vi "Day04-05_지진 계측기 프로젝트_생산자,소비자.vi"() -> ()   [LabVIEW 2021]
uses:
  <vilib>/numeric/Random Number (Range) DBL.vi
panel:
  out "웨이브폼 차트":dbl(graph)
  in  "알람 리셋":bool
  out "LED":bool
  in  "정지":bool
  in  "감지 시작":bool
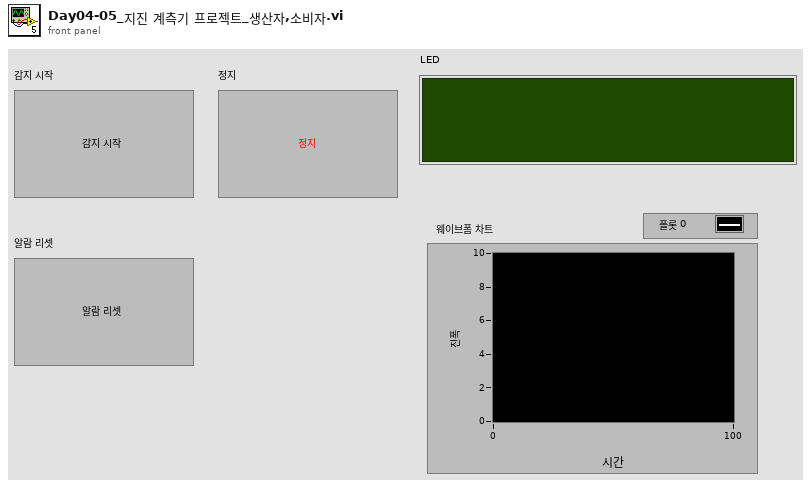
[diagram p1: front panel]
types:
  T1 = typedef "지진 계측기 상태 열거형 상수.ctl" = enum16{"초기화", "대기", "감지 시작", "알림 리셋", "정지"}
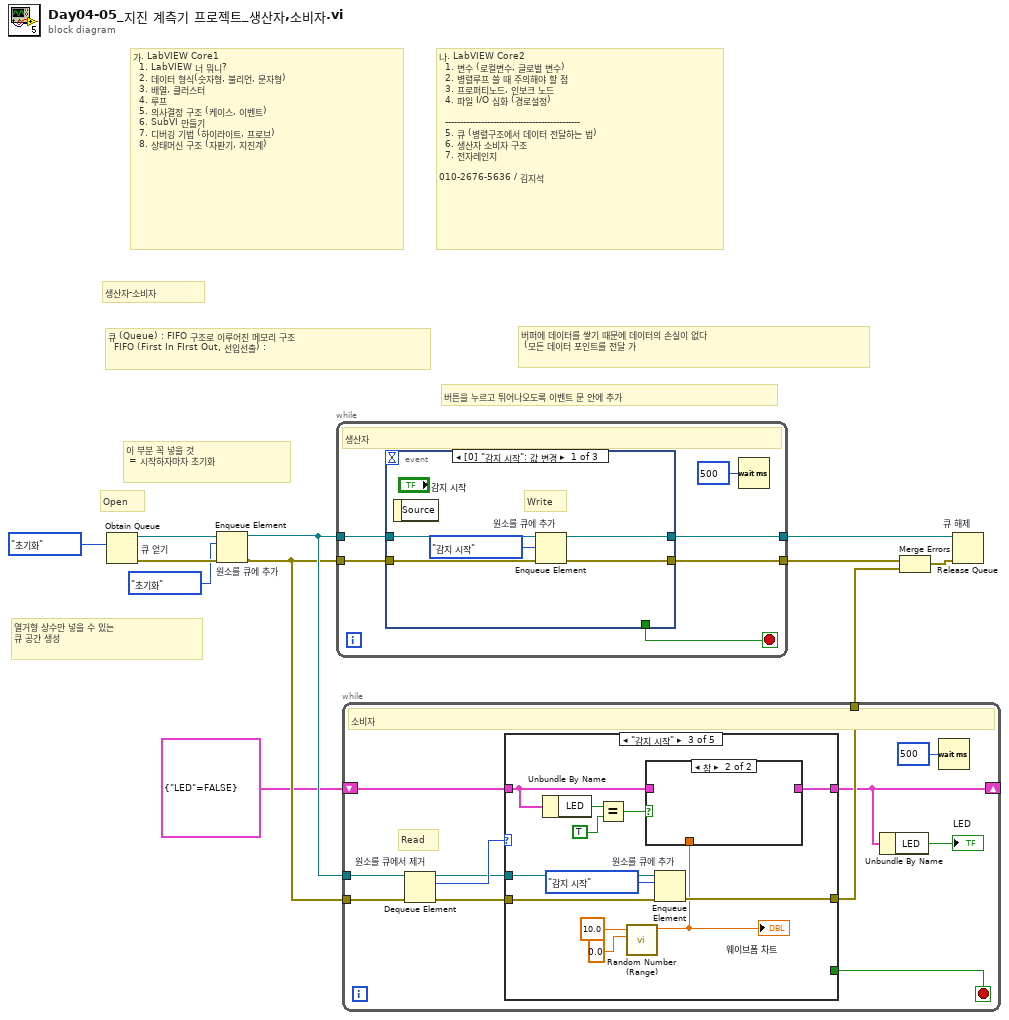
[diagram p0: block diagram]
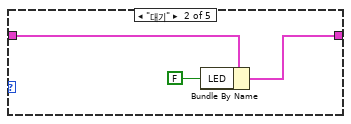
[diagram p3: hidden frame]
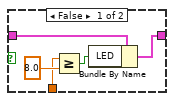
[diagram p4: hidden frame]
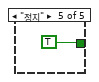
[diagram p6: hidden frame]
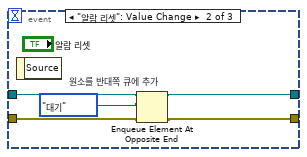
[diagram p7: hidden frame]
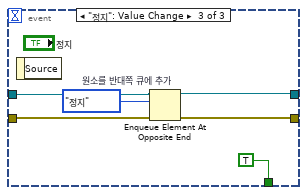
[diagram p8: hidden frame]
diagram:
  # "생산자-소비자"
  # "열거형 상수만 넣을 수 있는\n큐 공간 생성"
  # "이 부분 꼭 넣을 것\n = 시작하자마자 초기화"
  # "버튼을 누르고 튀어나오도록 이벤트 문 안에 추가"
  # "버퍼에 데이터를 쌓기 때문에 데이터의 손실이 없다\n (모든 데이터 포인트를 전달 가"
  # "Open"
  # "큐 (Queue) : FIFO 구조로 이루어진 메모리 구조\n  FIFO (First In FIrst Out, 선입선출) :"
  # "나. LabVIEW Core2\n  1. 변수 (로컬변수, 글로벌 변수)\n  2. 병렬루프 쓸 때 주의해야 할 점\n  3. 프로퍼티노드, 인보크 노드\n  4. 파일 I/O 심화 (경로설정)\n\n  ---------------------------------------------\n  5. 큐 (병렬구조에서 데이터 전달하는 법)\n  6. 생산자 소비자 구조\n  7. 전자레인지\n\n010-2676-5636 / 김지석"
  # "가. LabVIEW Core1\n  1. LabVIEW 너 뭐니?\n  2. 데이터 형식(숫자형, 불리언, 문자형)\n  3. 배열, 클러스터\n  4. 루프\n  5. 의사결정 구조 (케이스, 이벤트)\n  6. SubVI 만들기\n  7. 디버깅 기법 (하이라이트, 프로브)\n  8. 상태머신 구조 (자판기, 지진계)"
  n1 = Obtain Queue "큐 얻기"(element data type=지진_계측기_상태_열거형_상수."초기화") -> (queue out=w6:refnum<queue>, error out=w4:errorcluster)  [unwired: 4 in, 1 out]
  n2 = Enqueue Element "원소를 큐에 추가"(queue=w6, element=지진_계측기_상태_열거형_상수."초기화" ("원소"), error in (no error)=w4) -> (queue out=w5:refnum<queue>, error out=w3:errorcluster)  [unwired: 1 in, 1 out]
  n3 = while {
    tunnel: w5 -> [w17]
    tunnel: w3 -> [w16]
    tunnel: [w14] -> w8
    tunnel: [w13] -> w9
    stop <- w12 stop-if-true
    # "생산자"
    n4 = event shown="[0] \"감지 시작\": 값 변경" {
      selector: _ -> [_ _ _]
      dyn-events: _ -> [_ _ _]
      timeout: _ -> [_ _ _]
      tunnel: w17 -> [w22 w26 w30]
      tunnel: w16 -> [w19 w25 w31]
      tunnel: [w21 w27 w28] -> w14
      tunnel: [w20 w24 w32] -> w13
      tunnel: [_ _ TRUE] -> w12
      event "감지 시작": Value Change {
        # "Write"
        n5 = event-data() -> ()  [unwired: 1 in, 1 out]
        n6 = Enqueue Element "원소를 큐에 추가"(queue=w22, element=지진_계측기_상태_열거형_상수."감지 시작", error in (no error)=w19) -> (queue out=w21:refnum<queue>, error out=w20:errorcluster)  [unwired: 1 in, 1 out]
      }
      event "알람 리셋": Value Change {
        n7 = event-data() -> ()  [unwired: 1 in, 1 out]
        n8 = Enqueue Element At Opposite End "원소를 반대쪽 큐에 추가"(queue=w26, element=지진_계측기_상태_열거형_상수."대기", error in (no error)=w25) -> (queue out=w27:refnum<queue>, error out=w24:errorcluster)  [unwired: 1 in, 1 out]
      }
      event "정지": Value Change {
        n9 = event-data() -> ()  [unwired: 1 in, 1 out]
        n10 = Enqueue Element At Opposite End "원소를 반대쪽 큐에 추가"(queue=w30, element=지진_계측기_상태_열거형_상수."정지", error in (no error)=w31) -> (queue out=w28:refnum<queue>, error out=w32:errorcluster)  [unwired: 1 in, 1 out]
      }
    }
    n11 = Wait (ms)(milliseconds to wait=u32 500 ("대기 시간 (ms)")) -> ()  [unwired: 1 out]
  }
  n12 = while {
    tunnel: w3 -> [w44]
    tunnel: w5 -> [w43]
    tunnel: [w37] -> w10
    shift-right: [w34] -> _
    shift-left: cluster{"LED":bool} {"LED"=FALSE} -> [w35]
    stop <- w40 stop-if-true
    # "Read"
    # "소비자"
    n13 = Dequeue Element "원소를 큐에서 제거"(queue=w43, error in (no error)=w44) -> (queue out=w39:refnum<queue>, element=w41:T1, error out=w38:errorcluster)  [unwired: 1 in, 1 out]
    n14 = case shown="\"감지 시작\"" w41 {
      tunnel: [_ _ _ _ TRUE] -> w40
      tunnel: w39 -> [_ _ w59 _ _]
      tunnel: w38 -> [_ _ w58 _ _]
      tunnel: [_ _ w57 _ _] -> w37
      tunnel: w35 -> [_ w46 w49 _ _]
      tunnel: [_ w45 w53 _ _] -> w34
      frame "초기화", Default {
      }
      frame "대기" {
        n15 = Bundle By Name(cluster=w46, "LED"=FALSE) -> (w45:cluster{"LED":bool})
      }
      frame "감지 시작" {
        n16 = Unbundle By Name(w49) -> ("LED"=w54:bool)
        n17 = Equal?(x=w54, y=TRUE) -> (x = y?=w55:bool)
        n18 = call-poly <vilib>:"Random Number (Range).vi"("lower bound (0)"=0.0, "upper bound (100)"=10.0) -> ("number"=w48:dbl)  [unwired: 9 in]
        "웨이브폼 차트" <- w48
        n19 = case shown="참" w55 {
          tunnel: [w63 _] -> w53
          tunnel: w49 -> [w64 _]
          tunnel: w48 -> [w61 _]
          frame False {
            n20 = Greater Or Equal?(x=w61, y=8.0) -> (x >= y?=w60:bool)
            n21 = Bundle By Name(cluster=w64, "LED"=w60) -> (w63:cluster{"LED":bool})
          }
          frame True {
          }
        }
        n22 = Enqueue Element "원소를 큐에 추가"(queue=w59, element=지진_계측기_상태_열거형_상수."감지 시작", error in (no error)=w58) -> (error out=w57:errorcluster)  [unwired: 1 in, 2 out]
      }
      frame "알림 리셋" {
      }
      frame "정지" {
      }
    }
    n23 = Unbundle By Name(w34) -> ("LED"=→"LED":bool)
    n24 = Wait (ms)(milliseconds to wait=u32 500 ("대기 시간 (ms)")) -> ()  [unwired: 1 out]
  }
  n25 = Merge Errors(w9, w10) -> (w11:errorcluster)
  n26 = Release Queue "큐 해제"(queue=w8, error in (no error)=w11) -> ()  [unwired: 1 in, 3 out]
